vi "Initialize Transfers.vi"(7 "component name":string, 8 "error in":errorcluster, 10 "Labeled RX Transfer Configurations":T2(array[cluster]), 11 "Labeled TX Transfer Configurations":T2(array[cluster])) -> (0 "error out":errorcluster, 2 "max buffer size":i32 format="%d bytes", 3 "Labeled Transfer Parameters":T2(array[cluster]))   [LabVIEW 2020, in "RDMA.lvlib" / "RDMA Transceiver.lvclass"]
doc: "Initializes all transfers by creating the needed RDMA sessions"
uses:
  RDMA Transceiver.lvclass
  DSF Core.lvlibp/Classes/Configuration/Core/Transfer/Transfer Configuration.lvclass
  Transfer Parameters.ctl
  RDMA Transceiver.lvclass/RDMA Transceiver.ctl
  Throw Invalid RDMA Configuration Error.vi
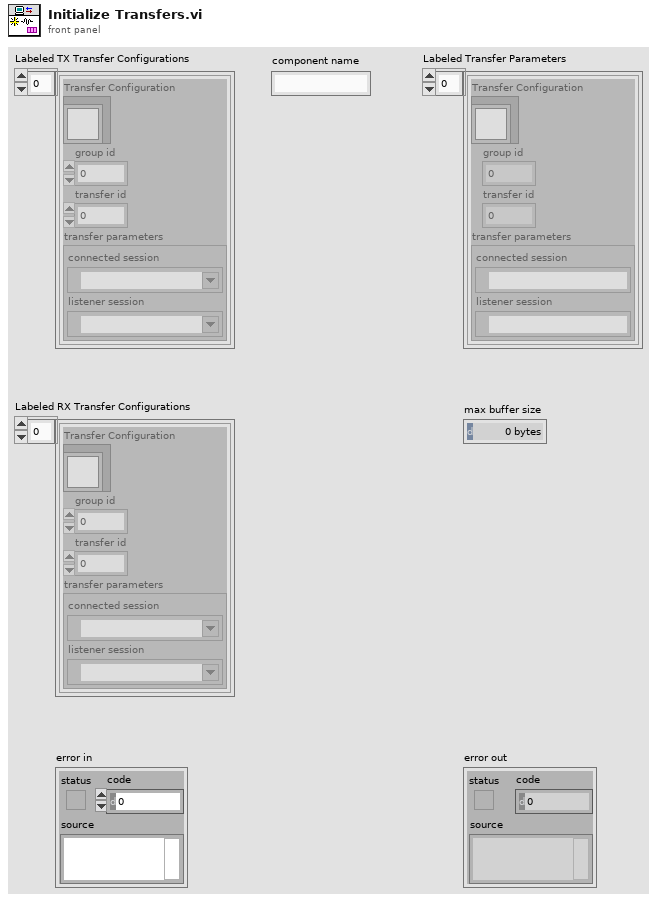
[diagram p1: front panel]
types:
  T1 = typedef "RDMA.lvlib/RDMA Transceiver.lvclass/Transfer Parameters.ctl" = cluster{"connected session":refnum<k21>, "listener session":refnum<k21>}
  T2 = cluster{"Transfer Configuration":refnum<class "Transfer Configuration.lvclass">, "group id":i32, "transfer id":i32, "transfer parameters":T1}[]
  T3 = cluster{"Transfer Configuration":refnum<class "Transfer Configuration.lvclass">, "group id":i32, "transfer id":i32, "transfer parameters":T1}
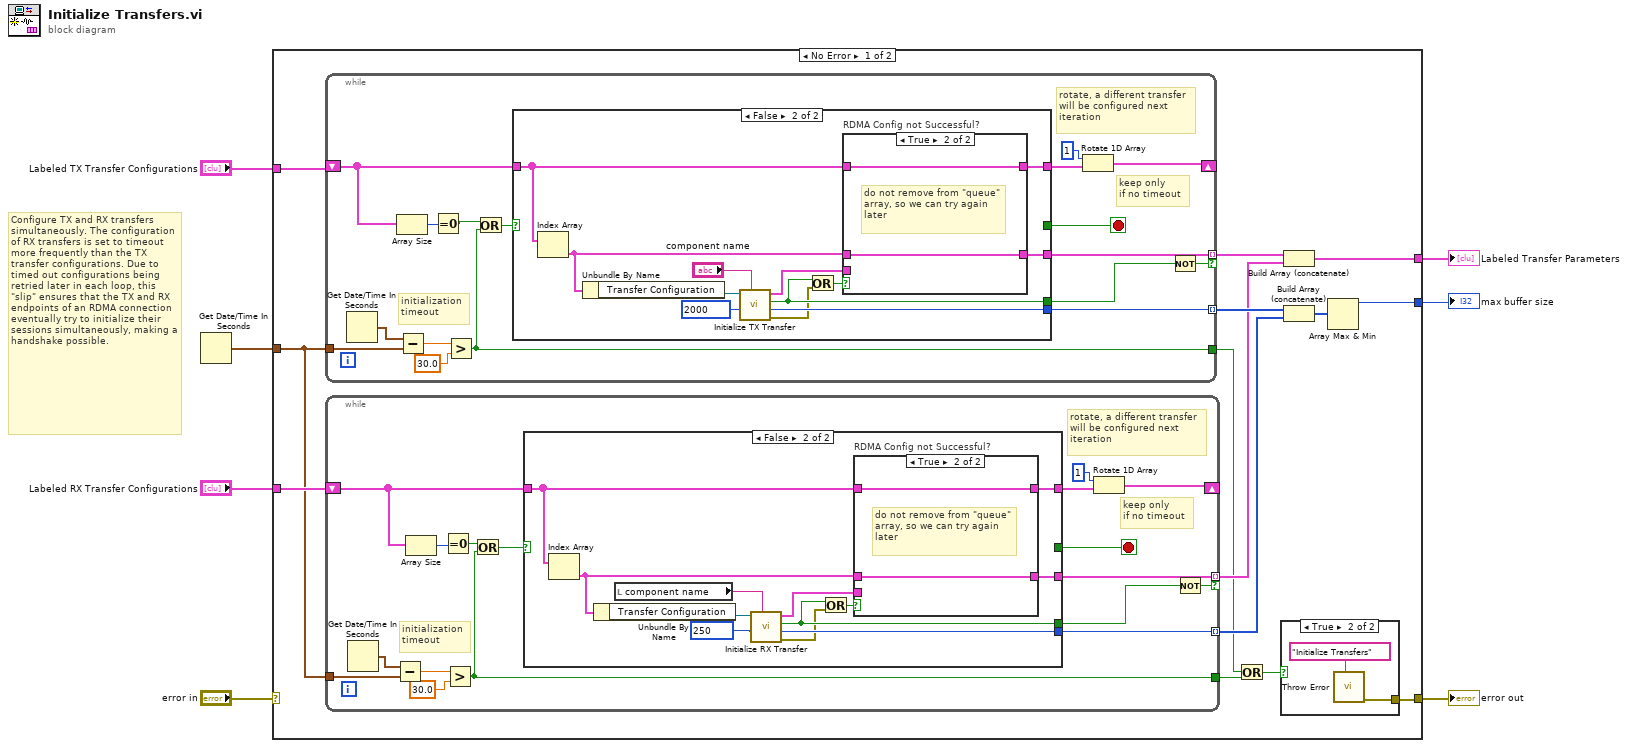
[diagram p0: block diagram]
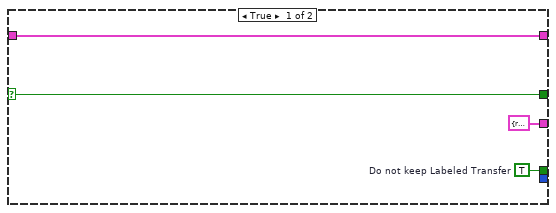
[diagram p2: hidden frame]
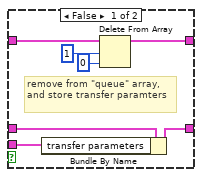
[diagram p3: hidden frame]
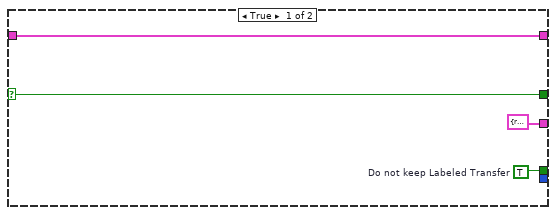
[diagram p4: hidden frame]
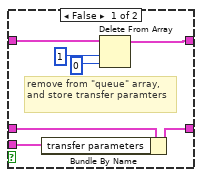
[diagram p5: hidden frame]
diagram:
  # "Configure TX and RX transfers simultaneously. The configuration of RX transfers is set to timeout more frequently than the TX transfer configurations. Due to timed out configurations being retried later in each loop, this \"slip\" ensures that the TX and RX endpoints of an RDMA connection eventually try to initialize their sessions simultaneously, making a handshake possible."
  n1 = Get Date/Time In Seconds() -> (seconds since 1Jan1904=w1:timestamp)
  n2 = case shown="No Error" "error in" {
    selector: "error in" -> [_ w108]
    tunnel: "Labeled TX Transfer Configurations" -> [w21 _]
    tunnel: [w11 w108] -> w6
    tunnel: [w17 _] -> w5
    tunnel: [w16 _] -> w4
    tunnel: "Labeled RX Transfer Configurations" -> [w15 _]
    tunnel: w1 -> [w10 _]
    frame No Error {
      n3 = while {
        shift-right: [w32] -> _
        shift-left: w21 -> [w36]
        tunnel: [w38] -> w20 mode=indexing if=w34
        tunnel: [w35] -> w19 mode=indexing
        tunnel: w10 -> [w26]
        tunnel: [w22] -> w8
        stop <- w30 stop-if-true
        # "initialization \ntimeout"
        # "keep only\nif no timeout"
        # "rotate, a different transfer will be configured next iteration"
        n4 = Get Date/Time In Seconds() -> (seconds since 1Jan1904=w27:timestamp)
        n5 = Array Size(array=w36) -> (size(s)=w25:i32)
        n6 = Subtract(x=w27, y=w26) -> (x-y=w28:dbl)
        n7 = Equal To 0?(x=w25) -> (x = 0?=w23:bool)
        n8 = Greater?(x=w28, y=30.0) -> (0:w22:bool)
        n9 = Or(x=w23, y=w22) -> (x .or. y?=w24:bool)
        n10 = case shown="False" w24 {
          selector: w24 -> [w39 _]
          tunnel: [T3 {"Transfer Configuration"=refnum, "group id"=0, "transfer id"=0, "transfer parameters"={"connected session"="", "listener session"=""}} ("cluster") w54] -> w38
          tunnel: [w40 w44] -> w37
          tunnel: w36 -> [w42 w52]
          tunnel: [w42 w50] -> w33
          tunnel: [_ w48] -> w35
          tunnel: [w39 _] -> w30
          frame True {
            w40 = TRUE  # Do not keep Labeled Transfer
          }
          frame False {
            n11 = Index Array(array=w52) -> (element=w51:T3)  [unwired: 1 in]
            n12 = Unbundle By Name(w51) -> ("Transfer Configuration"=w53:refnum<class "Transfer Configuration.lvclass">)
            n13 = call "Initialize TX Transfer.vi"("component name"="component name", "timeout (ms)"=2000, "Transfer Configuration in"=w53) -> ("error out"=w43:errorcluster, "buffer size"=w48:i32, "timeout?"=w44:bool, "transfer parameters"=w47:T1)  [unwired: 5 in]
            n14 = Or(x=w44, y=w43) -> (x .or. y?=w45:bool)
            n15 = case "RDMA Config not Successful?" shown="True" w45 {
              tunnel: w51 -> [w58 w62]
              tunnel: w47 -> [w61 _]
              tunnel: [w60 w62] -> w54
              tunnel: w52 -> [w57 w63]
              tunnel: [w59 w63] -> w50
              frame False {
                # "remove from \"queue\" array, and store transfer paramters"
                n16 = Bundle By Name(cluster=w58, "transfer parameters"=w61) -> (w60:T3)
                n17 = Delete From Array(array=w57, length=1, index=0 ("length")) -> (array with subset deleted=w59:T2)  [unwired: 1 out]
              }
              frame True {
                # "do not remove from \"queue\" array, so we can try again later"
              }
            }
          }
        }
        n18 = Rotate 1D Array(1:w33, 2:1 ("n")) -> (0:w32:T2)
        n19 = Not(x=w37) -> (.not. x?=w34:bool)
      }
      n20 = while {
        shift-right: [w74] -> _
        shift-left: w15 -> [w78]
        tunnel: [w80] -> w14 mode=indexing if=w76
        tunnel: [w77] -> w13 mode=indexing
        tunnel: w10 -> [w66]
        tunnel: [w65] -> w9
        stop <- w72 stop-if-true
        # "initialization \ntimeout"
        # "keep only\nif no timeout"
        # "rotate, a different transfer will be configured next iteration"
        n21 = Get Date/Time In Seconds() -> (seconds since 1Jan1904=w71:timestamp)
        n22 = Subtract(x=w71, y=w66) -> (x-y=w70:dbl)
        n23 = Array Size(array=w78) -> (size(s)=w69:i32)
        n24 = Equal To 0?(x=w69) -> (x = 0?=w68:bool)
        n25 = Greater?(x=w70, y=30.0) -> (0:w65:bool)
        n26 = Or(x=w68, y=w65) -> (x .or. y?=w67:bool)
        n27 = case shown="False" w67 {
          selector: w67 -> [w81 _]
          tunnel: [T3 {"Transfer Configuration"=refnum, "group id"=0, "transfer id"=0, "transfer parameters"={"connected session"="", "listener session"=""}} ("cluster") w96] -> w80
          tunnel: [w82 w86] -> w79
          tunnel: w78 -> [w84 w94]
          tunnel: [w84 w92] -> w75
          tunnel: [_ w91] -> w77
          tunnel: [w81 _] -> w72
          frame True {
            w82 = TRUE  # Do not keep Labeled Transfer
          }
          frame False {
            n28 = Index Array(array=w94) -> (element=w93:T3)  [unwired: 1 in]
            n29 = Unbundle By Name(w93) -> ("Transfer Configuration"=w95:refnum<class "Transfer Configuration.lvclass">)
            n30 = local read "component name"() -> (w89:string)
            n31 = call "Initialize RX Transfer.vi"("component name"=w89, "timeout (ms)"=250, "Transfer Configuration"=w95) -> ("error out"=w85:errorcluster, "buffer size"=w91:i32, "timeout?"=w86:bool, "transfer parameters"=w90:T1)  [unwired: 5 in]
            n32 = Or(x=w86, y=w85) -> (x .or. y?=w87:bool)
            n33 = case "RDMA Config not Successful?" shown="True" w87 {
              tunnel: w93 -> [w100 w104]
              tunnel: w90 -> [w103 _]
              tunnel: [w102 w104] -> w96
              tunnel: w94 -> [w99 w105]
              tunnel: [w101 w105] -> w92
              frame False {
                # "remove from \"queue\" array, and store transfer paramters"
                n34 = Bundle By Name(cluster=w100, "transfer parameters"=w103) -> (w102:T3)
                n35 = Delete From Array(array=w99, length=1, index=0 ("length")) -> (array with subset deleted=w101:T2)  [unwired: 1 out]
              }
              frame True {
                # "do not remove from \"queue\" array, so we can try again later"
              }
            }
          }
        }
        n36 = Rotate 1D Array(1:w75, 2:1 ("n")) -> (0:w74:T2)
        n37 = Not(x=w79) -> (.not. x?=w76:bool)
      }
      n38 = Or(x=w8, y=w9) -> (x .or. y?=w12:bool)
      n39 = case shown="True" w12 {
        tunnel: [_ w107] -> w11
        frame False {
        }
        frame True {
          n40 = call-poly "Throw Error.vi"("source vi name"="Initialize Transfers") -> ("error out"=w107:errorcluster)  [unwired: 10 in]
        }
      }
      n41 = Build Array (concatenate)(w20, w14) -> (w16:T2)
      n42 = Build Array (concatenate)(w19, w13) -> (w18:i32[])
      n43 = Array Max & Min(array=w18) -> (max value=w17:i32)  [unwired: 3 out]
    }
    frame Error {
    }
  }
  "error out" <- w6
  "Labeled Transfer Parameters" <- w4
  "max buffer size" <- w5
